vi "32_Temperature Simulator.vi"() -> ()   [LabVIEW 2018]
panel:
  in  "stop":bool
  out "Waveform Chart":dbl(graph)
  out "Temperature(C)":dbl
  in  "Upper temperature limit":dbl
  in  "Lower temperatue limit":dbl
  # "Develop a temperature simulator"
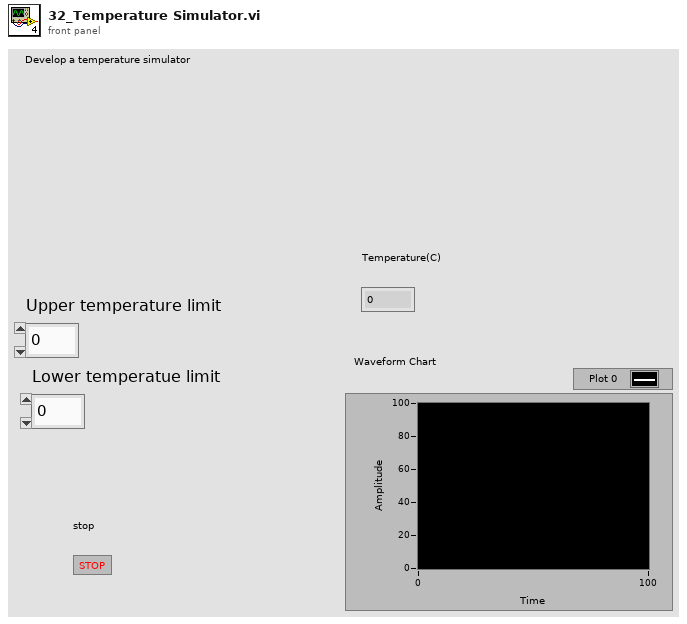
[diagram p1: front panel]
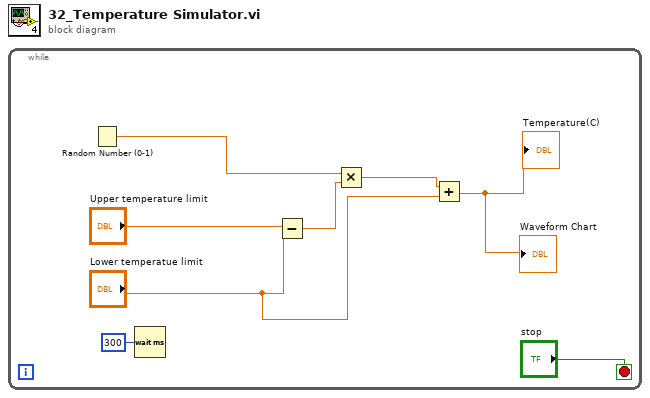
[diagram p0: block diagram]
diagram:
  n1 = while {
    stop <- "stop" stop-if-true
    n2 = Random Number (0-1)() -> (number: 0 to 1=w6:dbl)
    n3 = Wait (ms)(milliseconds to wait=u32 300) -> ()  [unwired: 1 out]
    n4 = Subtract(x="Upper temperature limit", y="Lower temperatue limit") -> (x-y=w5:dbl)
    n5 = Multiply(x=w6, y=w5) -> (x*y=w4:dbl)
    n6 = Add(x=w4, y="Lower temperatue limit") -> (x+y=→"Temperature(C)" →"Waveform Chart":dbl)
  }
